vi "string functions.vi"() -> ()   [LabVIEW 2018]
panel:
  in  "Boolean":bool
  in  "input 1":i32
  out "resulting string":string
  in  "initial string":string
  out "offset past match":i32
  out "before substring":string
  out "match substring":string
  out "after substring":string
  in  "offset (0) 4":i32
  in  "regular expression":string
  in  "string 4":string
  out "result string 2":string
  in  "offset (0) 3":i32
  in  "replace string (\"\")":string
  in  "input string":string
  in  "search string":string
  out "replaced substring":string
  out "result string":string
  in  "length (len. of substring)":i32
  in  "offset (0) 2":i32
  in  "substring (\"\")":string
  in  "string 3":string
  in  "length (rest)":i32
  in  "offset (0)":i32=3
  in  "string 2":string
  out "substring":string
  out "length":i32
  in  "string":string
  # "MATCH PATTERN"
  # "FORMAT INTO STRING"
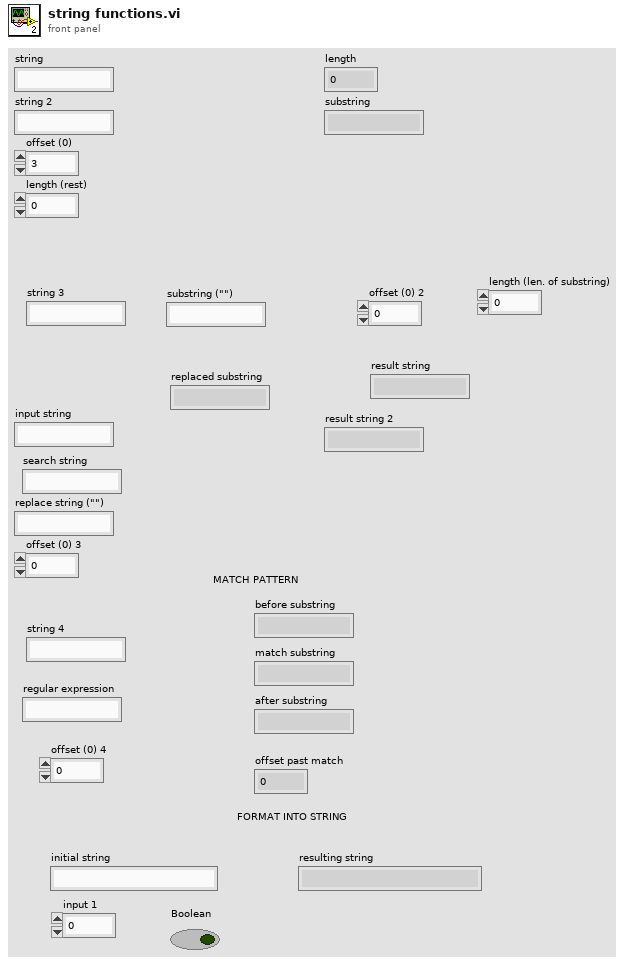
[diagram p1: front panel]
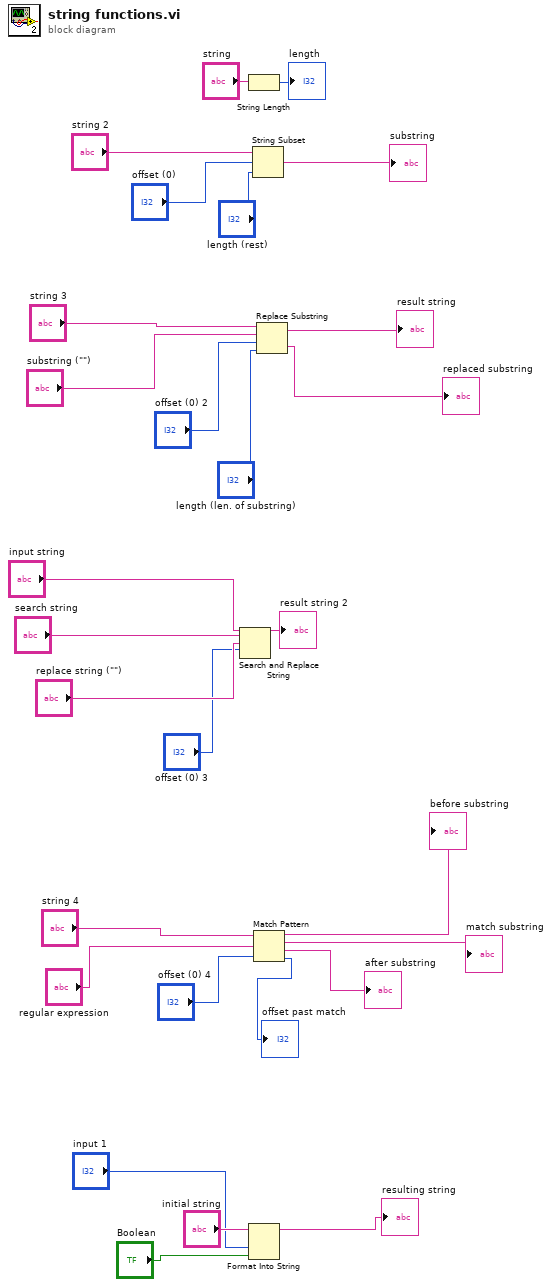
[diagram p0: block diagram]
diagram:
  n1 = Search and Replace String(input string="input string", search string="search string", replace string="replace string (\"\")", offset="offset (0) 3") -> (result string=→"result string 2":string)  [unwired: 4 in, 3 out]
  n2 = String Length(string="string") -> (length=→"length":i32)
  n3 = Format Into String "Format Into String"(initial string="initial string", "input 1", "Boolean") -> (resulting string=→"resulting string":string)  [unwired: 2 in, 1 out]
  n4 = String Subset(string="string 2", offset (0)="offset (0)", length (rest)="length (rest)") -> (substring=→"substring":string)
  n5 = Match Pattern(string="string 4", regular expression="regular expression", offset (0)="offset (0) 4") -> (before substring=→"before substring":string, match substring=→"match substring":string, after substring=→"after substring":string, offset past match=→"offset past match":i32)
  n6 = Replace Substring(2:"length (len. of substring)", 3:"offset (0) 2", 4:"substring (\"\")", 5:"string 3") -> (0:→"replaced substring":string, 1:→"result string":string)
